vi "Help Queue UI Control.vi"(8 "error In":errorcluster, 11 "UI_Top_Customer in":refnum<class "UI_Top_Customer.lvclass">) -> (0 "error out":errorcluster)   [LabVIEW 2021, in "UI_Top_Customer.lvclass"]
uses:
  UI_Top_Customer.lvclass
  UI_Top_Customer.lvclass/UI_Top_Customer.ctl
  <userlib>/John_Lib/Queue_Self/Queue_Self.lvlib
  <userlib>/John_Lib/AbstractActorTemplate/UIActorTop Messages/UI Initialize Msg/UI Initialize Msg.lvclass
  <userlib>/John_Lib/AbstractActorTemplate/UIActorTop Messages/UI Front Panel State Msg/UI Front Panel State Msg.lvclass
  <userlib>/John_Lib/Control/Panel State.ctl
  <vilib>/ActorFramework/Actor/Actor.lvclass
  C:/Program Files (x86)/National Instruments/LabVIEW 2021/user.lib/John_Lib/AbstractActorTemplate/AbstractActorTemplate/UIActorTop.lvclass
  C:/Program Files (x86)/National Instruments/LabVIEW 2021/vi.lib/ActorFramework/Actor/Actor.lvclass
  C:/Program Files (x86)/National Instruments/LabVIEW 2021/project/Create Actor from Template/_UI_Top_Customer/UI_Top_Customer.lvclass
  C:/Program Files (x86)/National Instruments/LabVIEW 2021/user.lib/John_Lib/Interfaces/FrontPanel Save Image/FrontPanel Save Image.lvclass
  C:/Program Files (x86)/National Instruments/LabVIEW 2021/user.lib/John_Lib/Interfaces/InsertMainSubPanel/InsertMainSubPanel.lvclass
panel:
  out "call chain":string[](array[string])
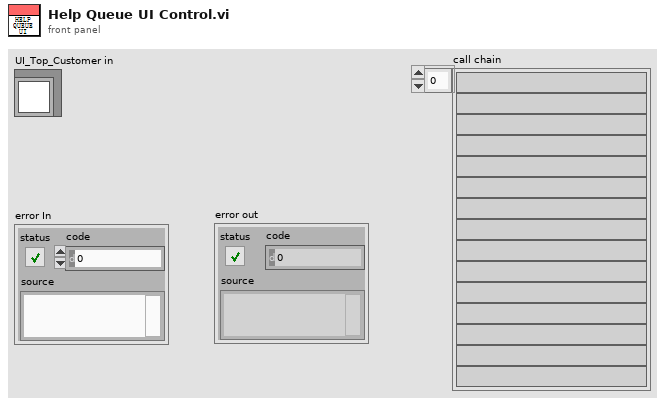
[diagram p1: front panel]
types:
  T1 = typedef "Panel State.ctl" = string
  T2 = typedef "LVRectTypeDef.ctl" = cluster{"Left":i16, "Top":i16, "Right":i16, "Bottom":i16}
  T3 = cluster{"button 1":bool, "button 2":bool, "button 3":bool, "button 4":bool}
  T4 = cluster{"Horizontal":i32, "Vertical":i32, "Scrolling":i32}
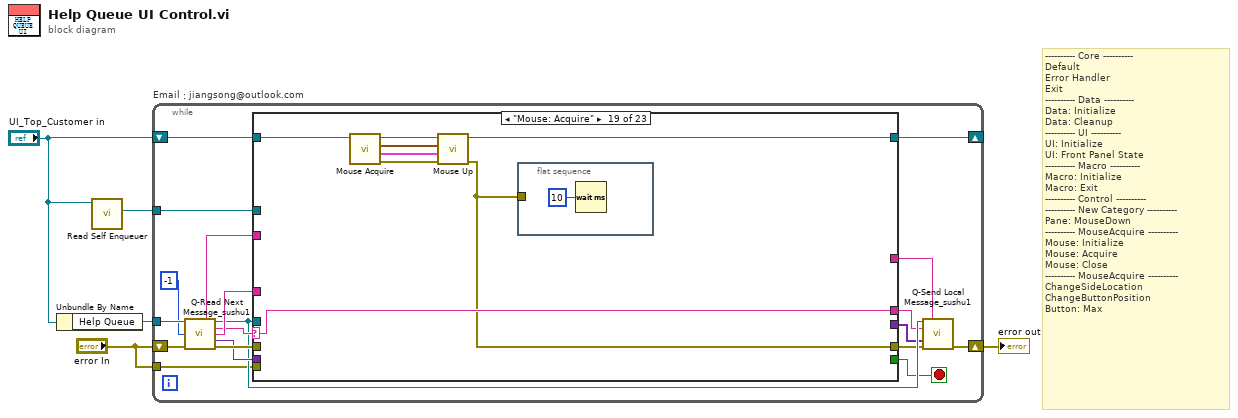
[diagram p0: block diagram]
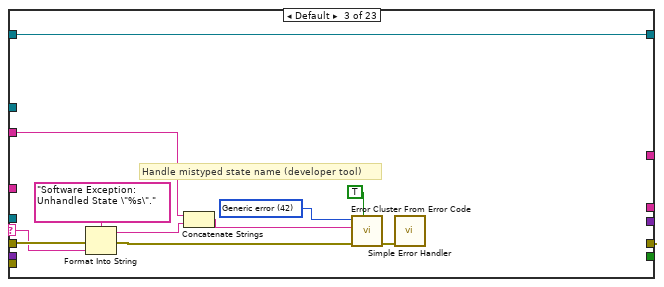
[diagram p4: hidden frame]
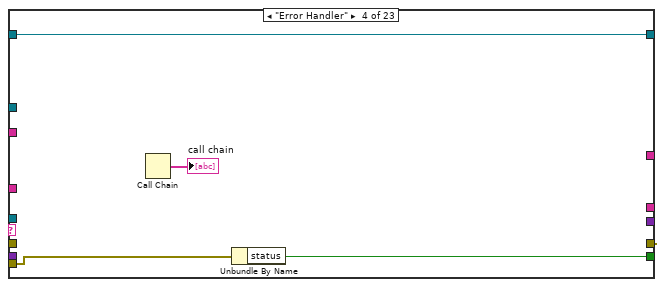
[diagram p5: hidden frame]
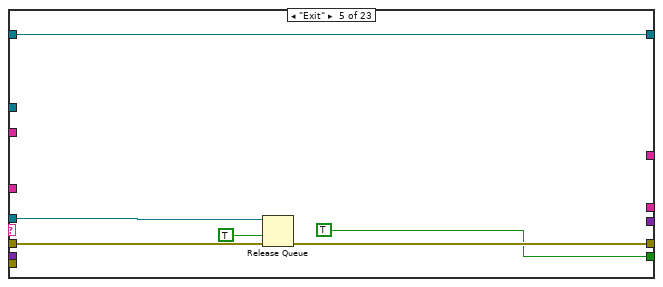
[diagram p6: hidden frame]
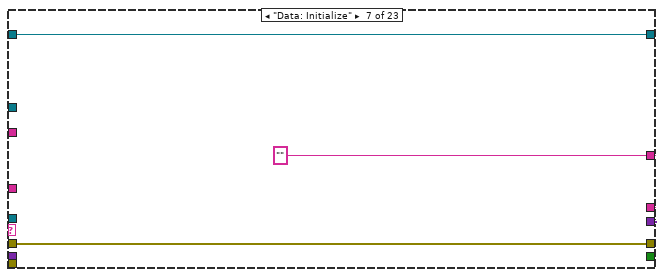
[diagram p8: hidden frame]
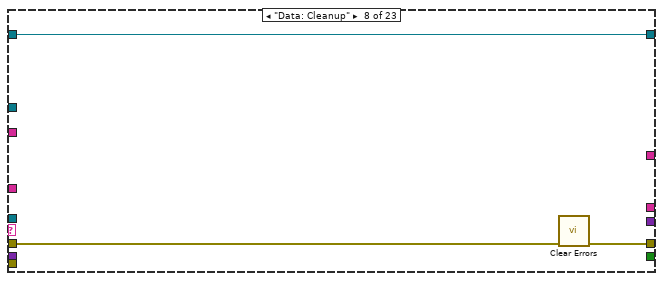
[diagram p9: hidden frame]
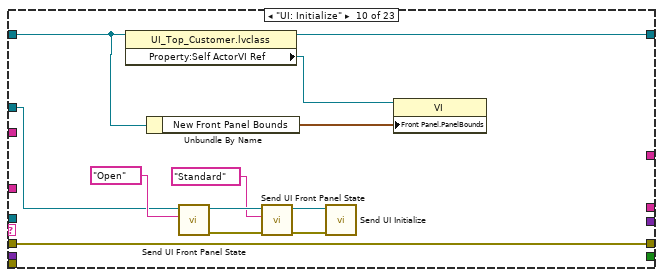
[diagram p11: hidden frame]
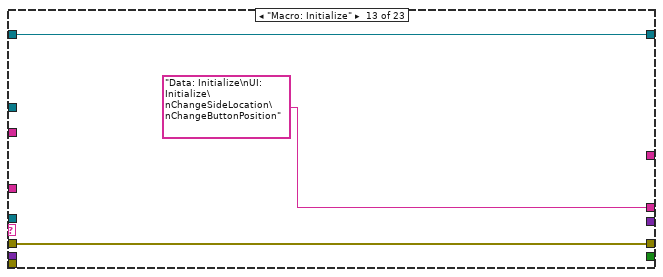
[diagram p14: hidden frame]
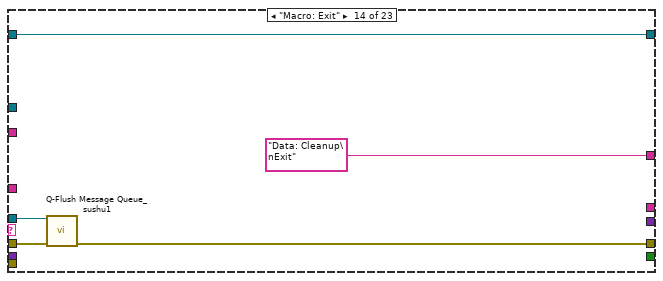
[diagram p15: hidden frame]
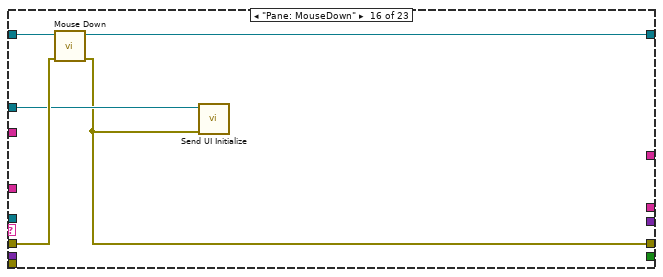
[diagram p17: hidden frame]
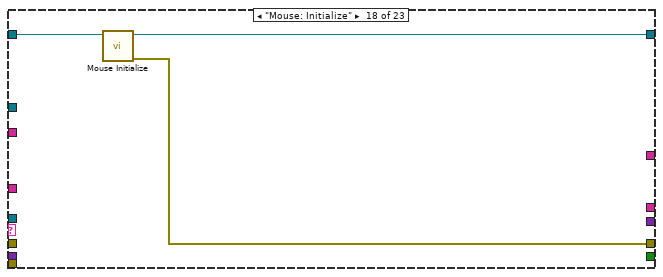
[diagram p19: hidden frame]
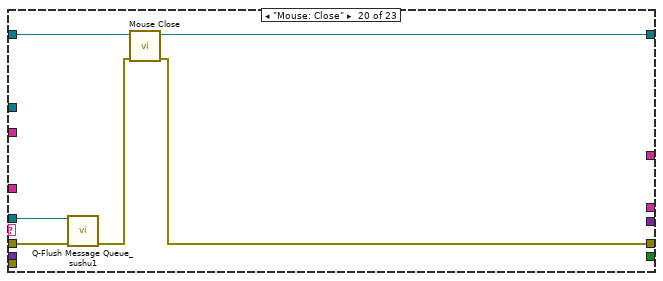
[diagram p20: hidden frame]
diagram:
  # "---------- Core ----------\nDefault\nError Handler\nExit\n---------- Data ----------\nData: Initialize\nData: Cleanup\n---------- UI ----------\nUI: Initialize\nUI: Front Panel State\n---------- Macro ----------\nMacro: Initialize\nMacro: Exit\n---------- Control ----------\n---------- New Category ----------\nPane: MouseDown\n---------- MouseAcquire ----------\nMouse: Initialize\nMouse: Acquire\nMouse: Close\n---------- MouseAcquire ----------\nChangeSideLocation\nChangeButtonPosition\nButton: Max"
  n1 = Unbundle By Name("UI_Top_Customer in") -> ("Help Queue"=w5:refnum<queue>)
  n2 = call <vilib>:"Read Self Enqueuer.vi"("Actor"="UI_Top_Customer in") -> ("Self Enqueuer"=w1:refnum<class "Message Enqueuer.lvclass">)  [unwired: 10 in]
  n3 = while "Email：jiangsong@outlook.com" {
    shift-right: [w13] -> w4
    shift-left: "error In" -> [w9]
    shift-right: [w24] -> _
    shift-left: "UI_Top_Customer in" -> [w11]
    tunnel: w5 -> [w10]
    tunnel: "error In" -> [w8]
    tunnel: w1 -> [w6]
    stop <- w12 stop-if-true
    n4 = call <userlib>:"Q-Read Next Message_sushu1.vi"("queue in"=w10, "timeout (1 ms)"=-1, "error in"=w9) -> ("Previous State + Arguments"=w22:string, "queue out"=w18:refnum<queue>, "Current State"=w19:string, "Arguments"=w21:string, "Data"=w20:variant, "error out"=w23:errorcluster)  [unwired: 6 in, 1 out]
    n5 = case shown="\"Mouse: Acquire\"" w19 {
      selector: w19 -> [_ _ w35 _ _ _ _ _ _ _ _ _ _ _ _ _ _ _ w106 _ _ _ _]
      tunnel: w18 -> [_ _ _ _ w49 _ _ _ _ _ _ _ _ w85 _ _ _ _ _ w111 _ _ _]
      tunnel: w20 -> [_ _ _ _ _ _ _ _ _ _ _ _ _ _ _ _ _ _ _ _ _ _ _]
      tunnel: [w25 w28 errorcluster {"status"=FALSE, "code"=0, "source"=""} ("error out") errorcluster {"status"=FALSE, "code"=0, "source"=""} ("error out") w47 w53 w58 w61 w63 w75 w76 w79 w81 w84 w89 w90 w96 w97 w100 w112 w116 w120 w123] -> w17
      tunnel: w23 -> [w25 w28 w36 _ w48 w53 w58 w59 w63 w75 w76 w79 w81 w86 w89 w92 w96 _ _ w110 w115 w119 _]
      tunnel: w11 -> [w26 w27 w30 w45 w51 w52 w57 w60 w62 w65 w77 w78 w82 w87 w88 w93 w95 w98 w107 w113 w117 w121 w124]
      tunnel: [w26 w27 w30 w45 w51 w52 w57 w60 w62 w66 w77 w78 w82 w87 w88 w94 w95 w99 w104 w114 w118 w122 w125] -> w24
      tunnel: w21 -> [_ _ _ _ _ _ _ _ _ _ _ _ _ _ _ _ _ _ _ _ _ _ _]
      tunnel: w22 -> [_ _ w29 _ _ _ _ _ _ _ _ _ _ _ _ _ _ _ _ _ _ _ _]
      tunnel: [_ _ _ _ _ _ w54 _ _ _ _ _ _ "Data: Cleanup\nExit" _ _ _ _ _ _ _ _ _] -> w14
      tunnel: [_ _ _ _ _ _ w54 _ _ _ _ _ "Data: Initialize\nUI: Initialize\nChangeSideLocation\nChangeButtonPosition" _ _ _ _ _ w106 _ _ _ _] -> w16
      tunnel: [_ _ _ _ _ _ w55 _ _ _ _ _ _ _ _ _ _ _ _ _ _ _ _] -> w15
      tunnel: [_ _ _ w42 TRUE _ _ _ _ _ _ _ _ _ _ _ _ _ _ _ _ _ _] -> w12
      tunnel: w8 -> [_ _ _ w43 _ _ _ _ _ _ _ _ _ _ _ _ _ _ _ _ _ _ _]
      tunnel: w6 -> [_ _ _ _ _ _ _ _ _ w64 _ _ _ _ _ w91 _ _ _ _ _ _ _]
      frame "", "Idle" {
        # "this actor is as the customer UI template\ndon't support message,\nso use queue process Action."
      }
      frame "---------- Core ----------" {
      }
      frame Default {
        w38 = 42 items=["No error", "Argument error", "Memory is full", "Out of zone", "End of file", "File already open", "Generic file I/O error", "File not found", "File permission error", "Disk is full", "Duplicate path", "Too many files open", "System feature not enabled", "Resource file not found", "Cannot add resource", "Resource not found", "Image not found", "Image memory error", "Pen does not exist", "Config type invalid", "Config token not found", "Config parse error", "Config memory error", "Bad external code format", "Bad external code offset", "External code not present", "Null window", "Destroy window error", "Null menu", "Print aborted", "Bad print record", "Print driver error", "Windows error during printing", "Memory error during printing", "Print dialog error", "Generic print error", "Invalid device refnum", "Device not found", "Device parameter error", "Device unit error", "Cannot open device", "Device call aborted", "Generic error", "Cancelled by user", "Object ID too low", "Object ID too high", "Object not in heap", "Unknown heap", "Unknown object (invalid DefProc)", "Unknown object (DefProc not in table)", "Message out of range", "Invalid (null) method", "Unknown message", "Manager call not supported", "Bad address", "Network operation in progress", "Network operation timed out", "Connection is busy", "Network attribute not supported", "Network error", "Address in use", "System out of memory", "Connection aborted", "Connection refused", "Not connected", "Already connected", "Connection closed", "Initialization error (interapplication manager)", "Bad occurrence", "Wait on unbound occurrence handler", "Occurrence queue overflow", "Datalog type conflict", "Unused", "Unrecognized type (interapplication manager)", "Memory corrupt", "Failed to make temporary DLL", "Old CIN version", "Drag socket not found", "Failed to load drop-object", "Failed to register OLE object", "Failed to release OLE object", "Format specifier type mismatch", "Unknown format specifier", "Too few format specifiers", "Too many format specifiers", "Scan failed", "Newer CIN version", "Error converting to variant", "Runtime menu error", "Password tampered", "Variant attribute not found", "Incompatible variant data type", "Event data is not available", "Event Store is not present", "Occurrence is not found", "Event Queue is not created", "Event info is not available", "Refnum passed is NULL", "Error retrieving Class GUID", "Error retrieving CoClass GUID", "Error retrieving TypeLib GUID.", "Bad built application magic bytes.", "Specific driver is different from the specific driver associated with the Logical Name.", "There is no session opened to the class driver.", "Max Error", "MAX - Error with config objects", "MAX - Error loading configuration", "MAX - Group not supported"]
        # "Handle mistyped state name (developer tool)"
        n6 = Format Into String(format string="Software Exception: Unhandled State \"%s\"." ("message"), error in=w36, w35) -> (resulting string=w32:string, error out=w39:errorcluster)  [unwired: 1 in]
        n7 = Concatenate Strings(w29, w32) -> (w31:string)
        n8 = call <vilib>:"Error Cluster From Error Code.vi"("show call chain? (False)"=TRUE, "error in (no error)"=w39, "error message (\"\")"=w31, "error code (0)"=w38) -> ("error out"=w34:errorcluster)  [unwired: 5 in]
        n9 = call <vilib>:"Simple Error Handler.vi"("error in (no error)"=w34) -> ()  [unwired: 4 in, 5 out]
      }
      frame "Error Handler" {
        # "Clear error"
        n10 = Call Chain() -> (call chain=→"call chain":string[])
        n11 = Unbundle By Name(w43) -> ("status"=w42:bool)
      }
      frame "Exit" {
        n12 = Release Queue(queue=w49, force destroy? (F)=TRUE, error in (no error)=w48) -> (error out=w47:errorcluster)  [unwired: 2 out]
      }
      frame "---------- Data ----------" {
      }
      frame "Data: Initialize" {
        w54 = "" ("Elements in Front")
        n13 = Build Array(variant ("Data")) -> (w55:variant[])
      }
      frame "Data: Cleanup" {
        n14 = call <vilib>:"Clear Errors.vi"("error in (no error)"=w59) -> ("error out"=w61:errorcluster)  [unwired: 5 in, 1 out]
      }
      frame "---------- UI ----------" {
      }
      frame "UI: Initialize" {
        n15 = property class="UI_Top_Customer.lvclass"(reference=w65) -> (reference out=w66:refnum<class "UI_Top_Customer.lvclass">, "Property:Self ActorVI Ref"=w67:refnum<vi>)  [unwired: 1 in, 1 out]
        n16 = Unbundle By Name(w65) -> ("New Front Panel Bounds"=w68:T2)
        n17 = call <userlib>:"Send UI Front Panel State.vi"("Argument"=T1 "Open", "Message Enqueuer"=w64) -> ("error out"=w69:errorcluster, "Message Enqueuer out"=w71:refnum<class "Message Enqueuer.lvclass">)  [unwired: 8 in]
        n18 = call <userlib>:"Send UI Front Panel State.vi"("error in (no error)"=w69, "Argument"=T1 "Standard", "Message Enqueuer"=w71) -> ("error out"=w74:errorcluster, "Message Enqueuer out"=w73:refnum<class "Message Enqueuer.lvclass">)  [unwired: 7 in]
        n19 = call <userlib>:"Send UI Initialize.vi"("error in (no error)"=w74, "Message Enqueuer"=w73) -> ()  [unwired: 8 in, 2 out]
        n20 = property class="VI"(reference=w67, "Front Panel.PanelBounds"=w68) -> ()  [unwired: 1 in, 2 out]
      }
      frame "UI: Front Panel State" {
      }
      frame "---------- Macro ----------" {
      }
      frame "Macro: Initialize" {
      }
      frame "Macro: Exit" {
        n21 = call <userlib>:"Q-Flush Message Queue_sushu1.vi"("queue in"=w85, "error in"=w86) -> ("error out"=w84:errorcluster)  [unwired: 11 in, 2 out]
      }
      frame "---------- Control ----------" {
      }
      frame "Pane: MouseDown" {
        n22 = call "Mouse Down.vi"("error in (no error)"=w92, "MainUI in"=w93) -> ("error out"=w90:errorcluster, "MainUI out"=w94:refnum<class "UI_Top_Customer.lvclass">)  [unwired: 8 in]
        n23 = call <userlib>:"Send UI Initialize.vi"("error in (no error)"=w90, "Message Enqueuer"=w91) -> ()  [unwired: 8 in, 2 out]
      }
      frame "---------- MouseAcquire ----------" {
      }
      frame "Mouse: Initialize" {
        n24 = call "Mouse Initialize.vi"("UI_Top_Customer in"=w98) -> ("error out"=w97:errorcluster, "UI_Top_Customer out"=w99:refnum<class "UI_Top_Customer.lvclass">)  [unwired: 9 in]
      }
      frame "Mouse: Acquire" {
        n25 = call "Mouse Acquire.vi"("UI_Top_Customer in"=w107) -> ("error out"=w103:errorcluster, "button info"=w101:T3, "axis info"=w102:T4, "UI_Top_Customer out"=w105:refnum<class "UI_Top_Customer.lvclass">)  [unwired: 7 in]
        n26 = call "Mouse Up.vi"("error in (no error)"=w103, "button info"=w101, "axis info"=w102, "UI_Top_Customer in"=w105) -> ("error out"=w100:errorcluster, "UI_Top_Customer out"=w104:refnum<class "UI_Top_Customer.lvclass">)  [unwired: 6 in]
        n27 = flat-sequence {
          tunnel: w100 -> [_]
          frame #0 {
            n28 = Wait (ms)(milliseconds to wait=u32 10 ("millisecond multiple")) -> ()  [unwired: 1 out]
          }
        }
      }
      frame "Mouse: Close" {
        n29 = call <userlib>:"Q-Flush Message Queue_sushu1.vi"("queue in"=w111, "error in"=w110) -> ("error out"=w109:errorcluster)  [unwired: 11 in, 2 out]
        n30 = call "Mouse Close.vi"("error in (no error)"=w109, "UI_Top_Customer in"=w113) -> ("error out"=w112:errorcluster, "UI_Top_Customer out"=w114:refnum<class "UI_Top_Customer.lvclass">)  [unwired: 8 in]
      }
      frame "ChangeSideLocation" {
        n31 = call "Side Location.vi"("error in (no error)"=w115, "UI_Top_Customer in"=w117) -> ("error out"=w116:errorcluster, "UI_Top_Customer out"=w118:refnum<class "UI_Top_Customer.lvclass">)  [unwired: 8 in]
      }
      frame "ChangeButtonPosition" {
        n32 = call "Change Buttons Position.vi"("error in (no error)"=w119, "MainUI in"=w121) -> ("error out"=w120:errorcluster, "MainUI out"=w122:refnum<class "UI_Top_Customer.lvclass">)  [unwired: 8 in]
      }
      frame "Button: Max" {
        n33 = call "Max Button Process.vi"("UI_Top_Customer in"=w124) -> ("error out"=w123:errorcluster, "UI_Top_Customer out"=w125:refnum<class "UI_Top_Customer.lvclass">)  [unwired: 9 in]
      }
    }
    n34 = call <userlib>:"Q-Send Local Message_sushu1.vi"("queue in"=w18, "Elements in Front"=w14, "Elements at Back"=w16, "message value"=w15, "error in"=w17) -> ("error out"=w13:errorcluster)  [unwired: 8 in, 2 out]
  }
  "error out" <- w4
